vi "SR_X_TCPReadBankCode.vi"(5 "address":string="192.168.0.101", 8 "BytesToRead":i32=147, 9 "BANK":string="01") -> (2 "CodeFound":bool, 3 "Code":string)   [LabVIEW 2023]
uses:
  <vilib>/Utility/error.llb/DialogType.ctl
panel:
  out "error out 3":errorcluster
  out "error out 2":errorcluster
  out "String lenght":i32
  out "All Codes":string
  out "bytes written":i32
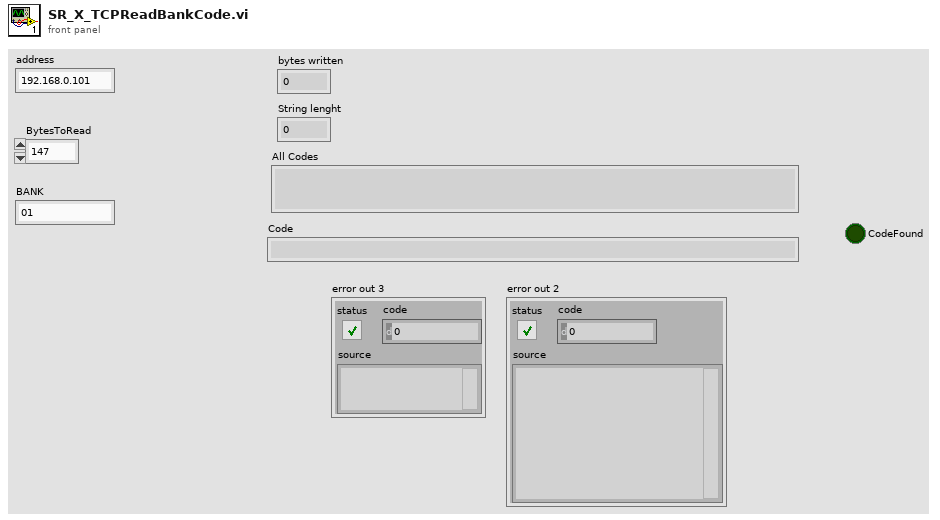
[diagram p1: front panel]
types:
  T1 = typedef "DialogType.ctl" = u16
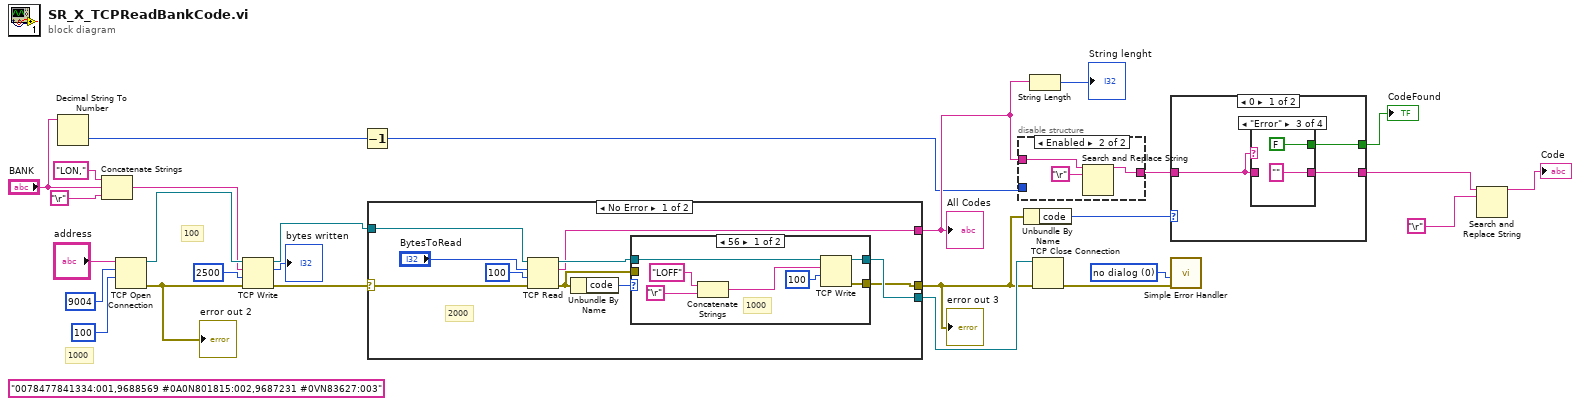
[diagram p0: block diagram]
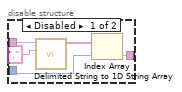
[diagram p2: hidden frame]
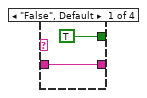
[diagram p3: hidden frame]
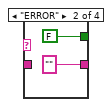
[diagram p4: hidden frame]
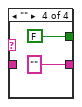
[diagram p5: hidden frame]
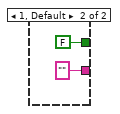
[diagram p6: hidden frame]
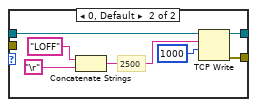
[diagram p7: hidden frame]
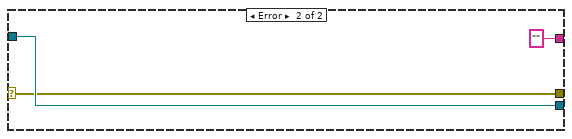
[diagram p8: hidden frame]
diagram:
  (unwired) "0078477841334:001,9688569 #0A0N801815:002,9687231 #0VN83627:003" ("String Data")
  w14 = T1 0 items=["no dialog", "OK message", "continue or stop message", "OK message + warnings", "continue/stop + warnings"] ("type of dialog (OK msg:1)")
  # "100"
  # "1000"
  n1 = Decimal String To Number(string="BANK") -> (number=w7:i32)  [unwired: 2 in, 1 out]
  n2 = Concatenate Strings("LON," ("data in"), "BANK", "\r") -> (w19:string)
  n3 = TCP Open Connection(address="address", remote port or service name=u16 9004, timeout ms (60000)=100) -> (connection ID=w23:refnum<k5>, error out=w24:errorcluster)  [unwired: 2 in]
  "error out 2" <- w24
  n4 = TCP Write(connection ID=w23, data in=w19, error in (no error)=w24, 9:2500 ("timeout ms (25000)")) -> (connection ID out=w18:refnum<k5>, bytes written=→"bytes written":i32, error out=w17:errorcluster)
  n5 = Decrement(x=w7) -> (x-1=w8:i32)
  n6 = case shown="No Error" w17 {
    selector: w17 -> [w36 w53]
    tunnel: w18 -> [w37 w54]
    tunnel: [w30 "" ("data out")] -> w10
    tunnel: [w32 w53] -> w6
    tunnel: [w33 w54] -> w16
    frame No Error {
      # "2000"
      n7 = TCP Read(connection ID=w37, bytes to read="BytesToRead", error in (no error)=w36, 9:100 ("timeout ms (25000)")) -> (connection ID out=w31:refnum<k5>, data out=w30:string, error out=w28:errorcluster)  [unwired: 1 in]
      n8 = Unbundle By Name(w28) -> ("code"=w34:i32)
      n9 = case shown="56" w34 {
        tunnel: [w44 w51] -> w33
        tunnel: [w43 w50] -> w32
        tunnel: w31 -> [w42 w49]
        tunnel: w28 -> [_ _]
        frame 56 {
          # "1000"
          n10 = Concatenate Strings("LOFF" ("data in"), "\r") -> (w39:string)
          n11 = TCP Write(connection ID=w42, data in=w39, 9:100 ("timeout ms (25000)")) -> (connection ID out=w44:refnum<k5>, error out=w43:errorcluster)  [unwired: 1 in, 1 out]
        }
        frame 0, Default {
          # "2500"
          n12 = Concatenate Strings("LOFF" ("data in"), "\r") -> (w46:string)
          n13 = TCP Write(connection ID=w49, data in=w46, 9:1000 ("timeout ms (25000)")) -> (connection ID out=w51:refnum<k5>, error out=w50:errorcluster)  [unwired: 1 in, 1 out]
        }
      }
    }
    frame Error {
    }
  }
  "All Codes" <- w10
  "error out 3" <- w6
  n14 = disable-structure shown="Enabled" {
    disable-tunnel: w10 -> [w59 w61]
    disable-tunnel: w8 -> [w57 _]
    disable-tunnel: [w55 w60] -> w4
    frame Disabled {
      n15 = call <vilib>:"Delimited String to 1D String Array.vi"("delimiter"=",", "delimited string"=w59) -> ("string array"=w58:string[])  [unwired: 9 in]
      n16 = Index Array(array=w58, index=w57) -> (element=w55:string)
    }
    frame Enabled {
      n17 = Search and Replace String(input string=w61, search string="\r") -> (result string=w60:string)  [unwired: 6 in, 3 out]
    }
  }
  n18 = Unbundle By Name(w6) -> ("code"=w5:i32)
  n19 = String Length(string=w10) -> (length=→"String lenght":i32)
  n20 = TCP Close Connection(connection ID=w16, error in (no error)=w6) -> (error out=w15:errorcluster)  [unwired: 1 in, 1 out]
  n21 = case shown="0" w5 {
    tunnel: [w64 "" ("AreaCode")] -> w3
    tunnel: [w65 FALSE ("AreaFound")] -> w9
    tunnel: w4 -> [w63 _]
    frame 0 {
      n22 = case shown="\"Error\"" w63 {
        tunnel: [TRUE FALSE FALSE FALSE] -> w65
        tunnel: [w66 "" "" ""] -> w64
        tunnel: w63 -> [w66 _ _ _]
        frame "False", Default {
        }
        frame "ERROR" {
        }
        frame "Error" {
        }
        frame "" {
        }
      }
    }
    frame 1, Default {
    }
  }
  "CodeFound" <- w9
  n23 = call <vilib>:"Simple Error Handler.vi"("type of dialog (OK msg:1)"=w14, "error in (no error)"=w15) -> ()  [unwired: 3 in, 5 out]
  n24 = Search and Replace String(input string=w3, search string="\r") -> (result string=→"Code":string)  [unwired: 6 in, 3 out]
